vi "ReadAnswer(Tab).vi"(0 "Bytes to Read":u32=10, 1 "Command (\\r is appended)":string="Q:", 2 "VRN IN":refnum<visa-resource-name>) -> (3 "error out":errorcluster, 4 "OKdone":bool, 5 "String Received":string, 6 "VRN OUT":refnum<visa-resource-name>)   [LabVIEW 2011]
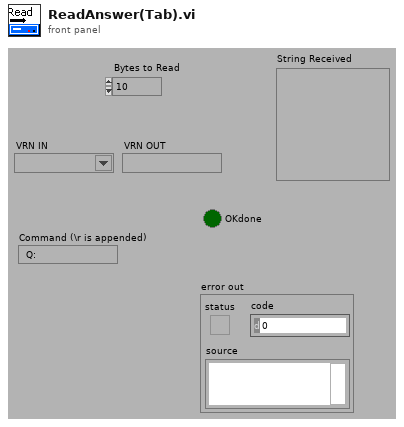
[diagram p1: front panel]
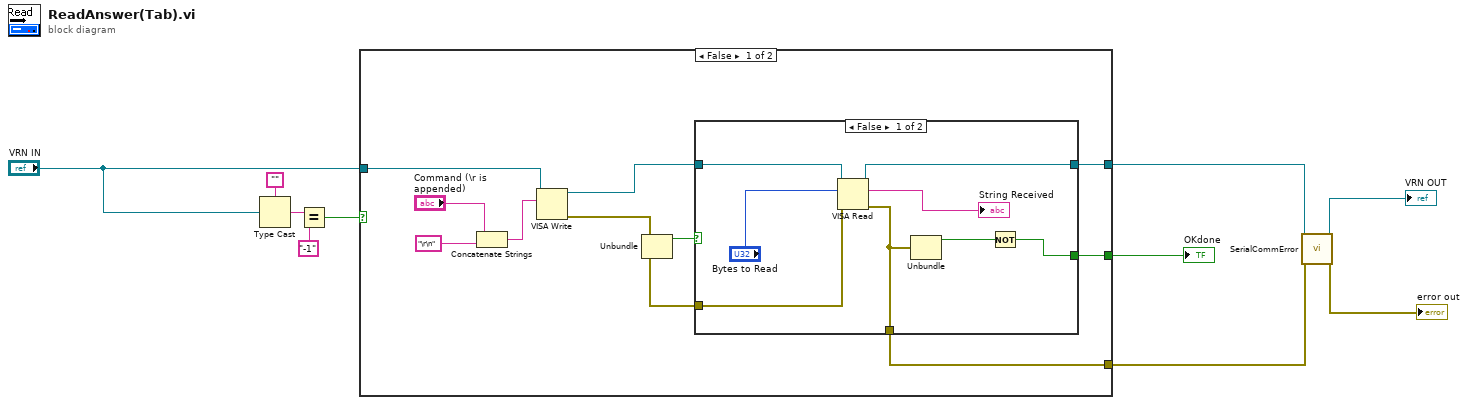
[diagram p0: block diagram]
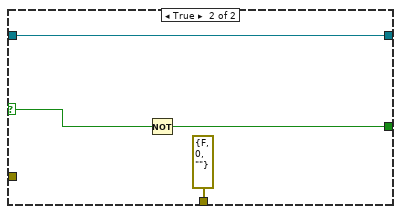
[diagram p2: hidden frame]
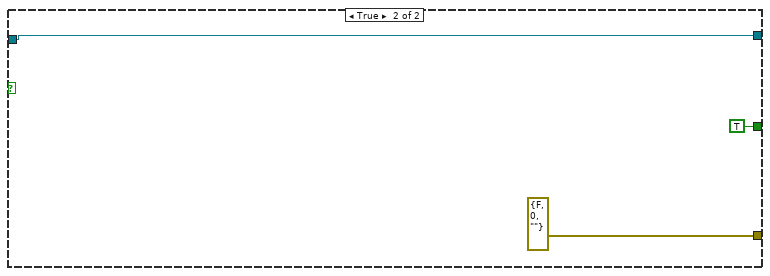
[diagram p3: hidden frame]
diagram:
  n1 = Type Cast(type="", x="VRN IN") -> (*(type *) &x=w8:string)
  n2 = Equal?(x=w8, y="-1") -> (x = y?=w6:bool)
  n3 = case shown="False" w6 {
    tunnel: [w18 TRUE] -> w10
    tunnel: "VRN IN" -> [w14 w34]
    tunnel: [w12 errorcluster {"status"=FALSE, "code"=0, "source"=""} ("error out")] -> w3
    tunnel: [w11 w34] -> w4
    frame False {
      n4 = Concatenate Strings("Command (\\r is appended)", "\r\n" ("string")) -> (w17:string)
      n5 = VISA Write(VISA resource name=w14, write buffer=w17) -> (VISA resource name out=w19:refnum<visa-resource-name>, error out=w13:errorcluster)  [unwired: 1 in, 1 out]
      n6 = Unbundle(w13) -> ("status"=w20:bool)  [unwired: 2 out]
      n7 = case shown="False" w20 {
        selector: w20 -> [_ w32]
        tunnel: w19 -> [w23 w29]
        tunnel: [w25 w31] -> w18
        tunnel: [w24 errorcluster {"status"=FALSE, "code"=0, "source"=""} ("error out")] -> w12
        tunnel: [w22 w29] -> w11
        tunnel: w13 -> [w21 _]
        frame False {
          n8 = VISA Read(VISA resource name=w23, byte count="Bytes to Read", error in (no error)=w21) -> (VISA resource name out=w22:refnum<visa-resource-name>, read buffer=→"String Received":string, error out=w24:errorcluster)  [unwired: 1 out]
          n9 = Unbundle(w24) -> ("status"=w27:bool)  [unwired: 2 out]
          n10 = Not(x=w27) -> (.not. x?=w25:bool)
        }
        frame True {
          n11 = Not(x=w32) -> (.not. x?=w31:bool)
        }
      }
    }
    frame True {
    }
  }
  "OKdone" <- w10
  n12 = call "SerialCommError.vi"("VISA IN"=w4, "error IN"=w3) -> ("VISA OUT"=→"VRN OUT":refnum<visa-resource-name>, "error OUT"=→"error out":errorcluster)  [unwired: 11 in, 1 out]
